vi "Open Pneumatics.vi"   [LabVIEW 2018]
uses:
  <vilib>/Rock Robotics/WPI/Solenoid/WPI_SolenoidChannel.ctl
  <vilib>/Rock Robotics/WPI/Solenoid/WPI_SolenoidOpenSingle.vi
types:
  T1 = typedef "WPI_SolenoidChannel.ctl" = enum8{"Solenoid 0", "Solenoid 1", "Solenoid 2", "Solenoid 3", "Solenoid 4", "Solenoid 5", "Solenoid 6", "Solenoid 7", "Invalid"}
  T2 = typedef "WPI_SolenoidDevRef.ctl" = cluster{"DevStatus":errorcluster, "Pneumatics Control Module":u8, "Forward Solenoid Channel":T1, "Reverse Solenoid Channel":T1}
  T3 = typedef "WPI_CompressorDevRef.ctl" = cluster{"DevStatus":errorcluster, "Pneumatics Control Module":u8}
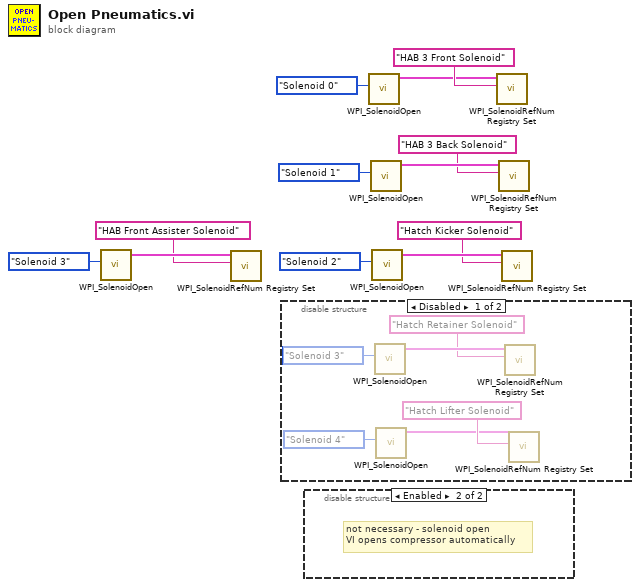
[diagram p0: block diagram]
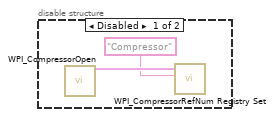
[diagram p3: hidden frame]
diagram:
  n1 = call-poly <vilib>:"WPI_SolenoidOpen.vi"("Solenoid Channel"=WPI_SolenoidChannel."Solenoid 3") -> ("SolenoidDevRef"=w3:T2)  [unwired: 9 in, 1 out]
  n2 = call <vilib>:"WPI_SolenoidRefNum Registry Set.vi"("refnum name"="HAB Front Assister Solenoid", "SolenoidDevRef"=w3) -> ()  [unwired: 8 in, 2 out]
  n3 = disable-structure shown="Disabled" {
    frame Disabled {
      n4 = call-poly <vilib>:"WPI_SolenoidOpen.vi"("Solenoid Channel"=WPI_SolenoidChannel."Solenoid 3") -> ("SolenoidDevRef"=w15:T2)  [unwired: 9 in, 1 out]
      n5 = call-poly <vilib>:"WPI_SolenoidOpen.vi"("Solenoid Channel"=WPI_SolenoidChannel."Solenoid 4") -> ("SolenoidDevRef"=w17:T2)  [unwired: 9 in, 1 out]
      n6 = call <vilib>:"WPI_SolenoidRefNum Registry Set.vi"("refnum name"="Hatch Retainer Solenoid", "SolenoidDevRef"=w15) -> ()  [unwired: 8 in, 2 out]
      n7 = call <vilib>:"WPI_SolenoidRefNum Registry Set.vi"("refnum name"="Hatch Lifter Solenoid", "SolenoidDevRef"=w17) -> ()  [unwired: 8 in, 2 out]
    }
    frame Enabled {
    }
  }
  n8 = disable-structure shown="Enabled" {
    frame Disabled {
      n9 = call <vilib>:"WPI_CompressorOpen.vi"() -> ("CompressorDevRef"=w20:T3)  [unwired: 14 in, 1 out]
      n10 = call <vilib>:"WPI_CompressorRefNum Registry Set.vi"("refnum name"="Compressor", "CompressorDevRef"=w20) -> ()  [unwired: 8 in, 2 out]
    }
    frame Enabled {
      # "not necessary - solenoid open\nVI opens compressor automatically"
    }
  }
  n11 = call-poly <vilib>:"WPI_SolenoidOpen.vi"("Solenoid Channel"=WPI_SolenoidChannel."Solenoid 0") -> ("SolenoidDevRef"=w4:T2)  [unwired: 9 in, 1 out]
  n12 = call-poly <vilib>:"WPI_SolenoidOpen.vi"("Solenoid Channel"=WPI_SolenoidChannel."Solenoid 1") -> ("SolenoidDevRef"=w9:T2)  [unwired: 9 in, 1 out]
  n13 = call-poly <vilib>:"WPI_SolenoidOpen.vi"("Solenoid Channel"=WPI_SolenoidChannel."Solenoid 2") -> ("SolenoidDevRef"=w12:T2)  [unwired: 9 in, 1 out]
  n14 = call <vilib>:"WPI_SolenoidRefNum Registry Set.vi"("refnum name"="HAB 3 Front Solenoid", "SolenoidDevRef"=w4) -> ()  [unwired: 8 in, 2 out]
  n15 = call <vilib>:"WPI_SolenoidRefNum Registry Set.vi"("refnum name"="HAB 3 Back Solenoid", "SolenoidDevRef"=w9) -> ()  [unwired: 8 in, 2 out]
  n16 = call <vilib>:"WPI_SolenoidRefNum Registry Set.vi"("refnum name"="Hatch Kicker Solenoid", "SolenoidDevRef"=w12) -> ()  [unwired: 8 in, 2 out]
